vi "AlliGator Quit Source Image ROI Manager.vi"(8 "Error In":errorcluster) -> (0 "Error Out":errorcluster)   [LabVIEW 2021, in "AlliGator ROIs.lvlib"]
doc: "Handles Source Image ROI manager quit event."
uses:
  AlliGator ROIs.lvlib
  AlliGator Source Image ROI Manager.vi
panel:
  # "see the AlliGator License on the block diagram (Ctrl+E or Window:Show Block Diagram)"
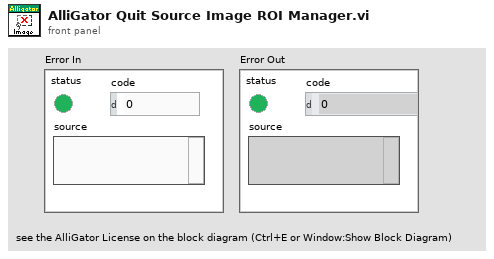
[diagram p1: front panel]
types:
  T1 = enum32{"Invalid", "Standard", "Closed", "Hidden", "Minimized", "Maximized"}
  T2 = typedef "AlliGator ROIs.lvlib/AlliGator Image ROI Event refnum.ctl" = refnum<user-event>
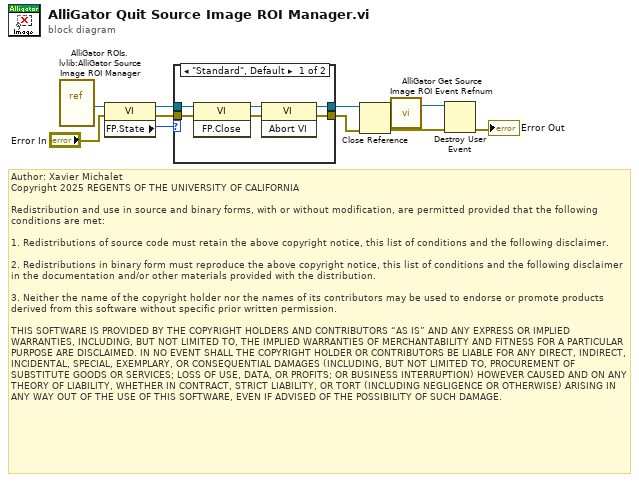
[diagram p0: block diagram]
diagram:
  # "Author: Xavier Michalet\nCopyright 2025 REGENTS OF THE UNIVERSITY OF CALIFORNIA\n\nRedistribution and use in source and binary forms, with or without modification, are permitted provided that the following conditions are met:\n\n1. Redistributions of source code must retain the above copyright notice, this list of conditions and the following disclaimer.\n\n2. Redistributions in binary form must reproduce the above copyright notice, this list of conditions and the following disclaimer in the documentation and/or other materials provided with the distribution.\n\n3. Neither the name of the copyright holder nor the names of its contributors may be used to endorse or promote products derived from this software without specific prior written permission.\n\nTHIS SOFTWARE IS PROVIDED BY THE COPYRIGHT HOLDERS AND CONTRIBUTORS “AS IS” AND ANY EXPRESS OR IMPLIED WARRANTIES, INCLUDING, BUT NOT LIMITED TO, THE IMPLIED WARRANTIES OF MERCHANTABILITY AND FITNESS FOR A PARTICULAR PURPOSE ARE DISCLAIMED. IN NO EVENT SHALL THE COPYRIGHT HOLDER OR CONTRIBUTORS BE LIABLE FOR ANY DIRECT, INDIRECT, INCIDENTAL, SPECIAL, EXEMPLARY, OR CONSEQUENTIAL DAMAGES (INCLUDING, BUT NOT LIMITED TO, PROCUREMENT OF SUBSTITUTE GOODS OR SERVICES; LOSS OF USE, DATA, OR PROFITS; OR BUSINESS INTERRUPTION) HOWEVER CAUSED AND ON ANY THEORY OF LIABILITY, WHETHER IN CONTRACT, STRICT LIABILITY, OR TORT (INCLUDING NEGLIGENCE OR OTHERWISE) ARISING IN ANY WAY OUT OF THE USE OF THIS SOFTWARE, EVEN IF ADVISED OF THE POSSIBILITY OF SUCH DAMAGE."
  n1 = vi-ref "AlliGator ROIs.lvlib:AlliGator Source Image ROI Manager.vi"() -> (w10:refnum<vi>)
  n2 = property class="VI"(reference=w10, error in="Error In") -> (reference out=w9:refnum<vi>, error out=w7:errorcluster, "FP.State"=w8:T1)
  n3 = case shown="\"Standard\", Default" w8 {
    tunnel: w9 -> [w15 w17]
    tunnel: w7 -> [w14 w18]
    tunnel: [w12 w18] -> w5
    tunnel: [w11 w17] -> w6
    frame "Standard", Default {
      n4 = invoke class="VI" method="FP.Close"(reference=w15, error in=w14) -> (reference out=w16:refnum<vi>, error out=w13:errorcluster)  [unwired: 1 in, 1 out]
      n5 = invoke class="VI" method="Abort VI"(reference=w16, error in=w13) -> (reference out=w11:refnum<vi>, error out=w12:errorcluster)  [unwired: 1 in, 1 out]
    }
    frame "Invalid", "Closed" {
    }
  }
  n6 = Close Reference(reference=w6, error in (no error)=w5) -> (error out=w2:errorcluster)
  n7 = call "AlliGator Get Source Image ROI Event Refnum.vi"() -> ("Source Image ROI Event Refnum"=w4:T2)
  n8 = Destroy User Event(user event=w4, error in=w2) -> (error out=→"Error Out":errorcluster)
